vi "Pump Currents Global.vi"() -> ()   [LabVIEW 2013]
panel:
  out "Pump Currents":fxp<+/-,28,17>[](array[numeric])
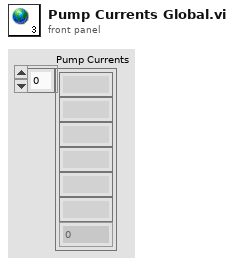
[diagram p1: front panel]
diagram:
